vi "Read Attributes.vi"(11 "New Data Msg":refnum<class "New Data Msg.lvclass">) -> (2 "Payload":cluster{"Data":string})   [LabVIEW 2025, in "Test_Nested.lvlib" / "New Data Msg.lvclass"]
uses:
  New Data Msg.lvclass
  New Data Msg.lvclass/New Data Msg.ctl
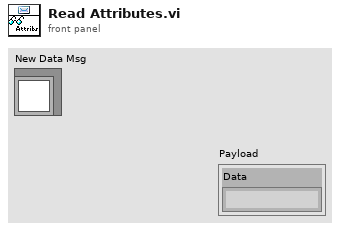
[diagram p1: front panel]
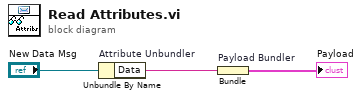
[diagram p0: block diagram]
diagram:
  n1 = Unbundle By Name "Attribute Unbundler"("New Data Msg") -> ("Data"=w1:string)
  n2 = Bundle "Payload Bundler"("Data"=w1) -> (→"Payload":cluster{"Data":string})  [unwired: 1 in]
